vi "MagX Get Ranged Info.vi"(4 "Save cache":bool, 5 "Station":string="Cell_3", 6 "Update experiment info file":bool, 7 "Use cache":bool=TRUE, 8 "error in":errorcluster, 9 "Day/time":timestamp, 10 "Days range":dbl=90.0, 11 "Hub URL":string="magx.lanl.gov") -> (0 "error out":errorcluster, 1 "resulting string":string, 2 "Online":bool, 3 "Data out":T1[](array[typedef]))   [LabVIEW 2024]
uses:
  Experiment info.ctl
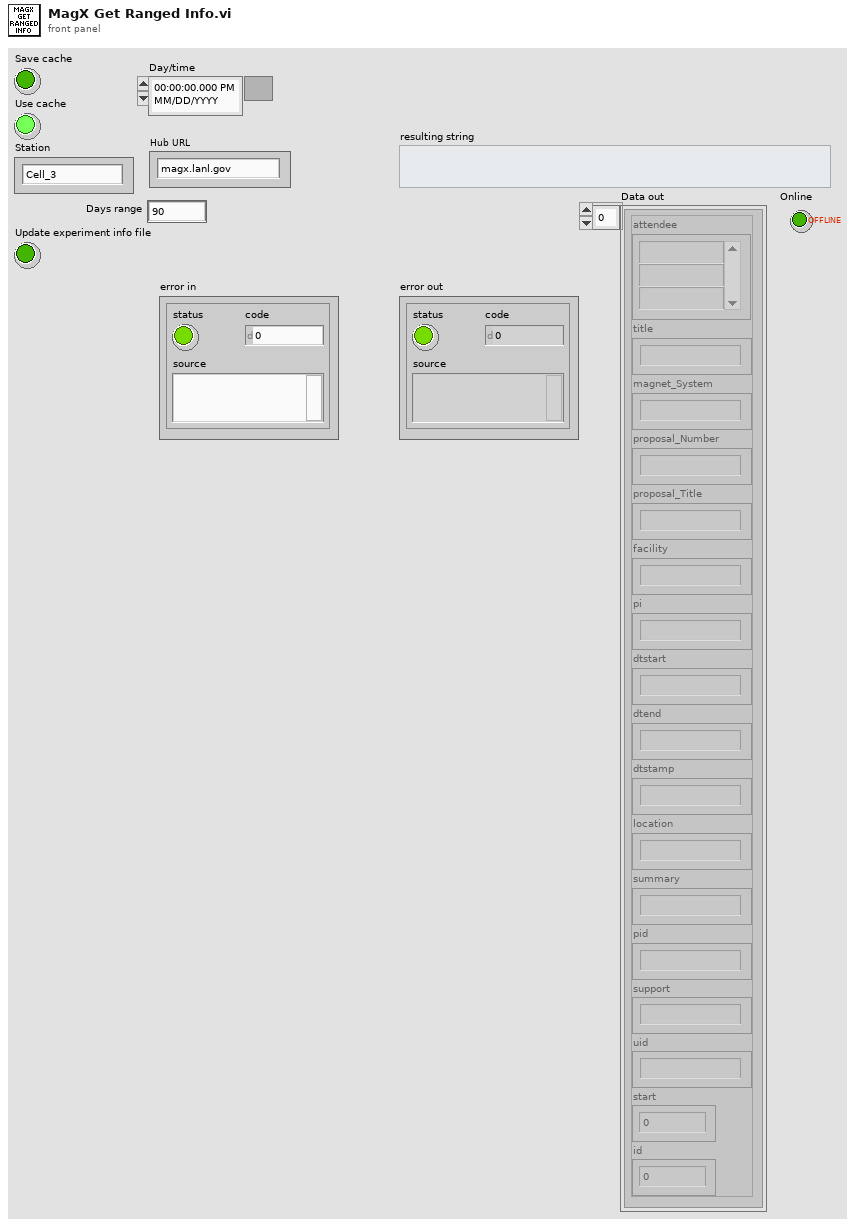
[diagram p1: front panel]
types:
  T1 = typedef "Experiment info.ctl" = cluster{"attendee":string[], "title":string, "magnet_System":string, "proposal_Number":string, "proposal_Title":string, "facility":string, "pi":string, "dtstart":string, "dtend":string, "dtstamp":string, "location":string, "summary":string, "pid":string, "support":string, "uid":string, "start":u64, "id":u64}
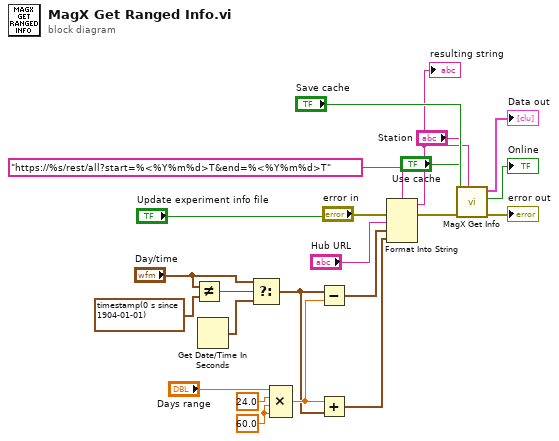
[diagram p0: block diagram]
diagram:
  w18 = 60.0
  n1 = Not Equal?(x="Day/time", y=timestamp(0 s since 1904-01-01) ("Day/time")) -> (x != y?=w9:bool)
  n2 = Get Date/Time In Seconds() -> (seconds since 1Jan1904=w7:timestamp)
  n3 = Select(t="Day/time", s=w9, f=w7) -> (s? t:f=w6:timestamp)
  n4 = Compound Arithmetic op=MULTIPLY("Days range", 24.0, w18, w18) -> (w21:dbl)
  n5 = Subtract(x=w6, y=w21) -> (x-y=w22:timestamp)
  n6 = Add(x=w21, y=w6) -> (x+y=w23:timestamp)
  n7 = Format Into String(format string="https://%s/rest/all?start=%<%Y%m%d>T&end=%<%Y%m%d>T", error in="error in", "Hub URL", w22, w23) -> (resulting string=w4:string, error out=w14:errorcluster)  [unwired: 1 in]
  "resulting string" <- w4
  n8 = call "MagX Get Info.vi"("Update experiment info file"="Update experiment info file", "url"=w4, "error in"=w14, "Save cache"="Save cache", "Use cache"="Use cache", "Station"="Station") -> ("error out"=→"error out":errorcluster, "Online"=→"Online":bool, "Data out"=→"Data out":T1[])  [unwired: 3 in]
